vi "GUI_laptop v5.vi"() -> ()   [LabVIEW 2019]
uses:
  <vilib>/Platform/TimedLoop/XDataNode/timing_clust.ctl
  <vilib>/Platform/TimedLoop/XDataNode/nitl_modes.ctl
  <vilib>/Platform/TimedLoop/XDataNode/wakeup.ctl
  <vilib>/Instr/_visa.llb/VISA Configure Serial Port (Instr).vi
  <vilib>/Utility/file.llb/Write Delimited Spreadsheet (DBL).vi
  <vilib>/platform/TimedLoop/XDataNode/XDataNode.xnode
  <vilib>/Platform/TimedLoop/XDataNode/XDNodeRunTimeDep.lvlib
panel:
  out "Array - Numeric":dbl[](array[numeric])
  out "Num bytes received":i32
  in  "Joystick Type":dbl(ring) items=["Rigid Joystick", "Free Joystick"]
  out "Finished Late? [i-1]":bool
  out "Iteration Duration":i64
  in  "Stop":bool
  in  "Save  Data":bool
  in  "Save Path":path
  out "error out":errorcluster
  in  "baud rate":u32=115200
  in  "VISA resource name":refnum<visa-resource-name>
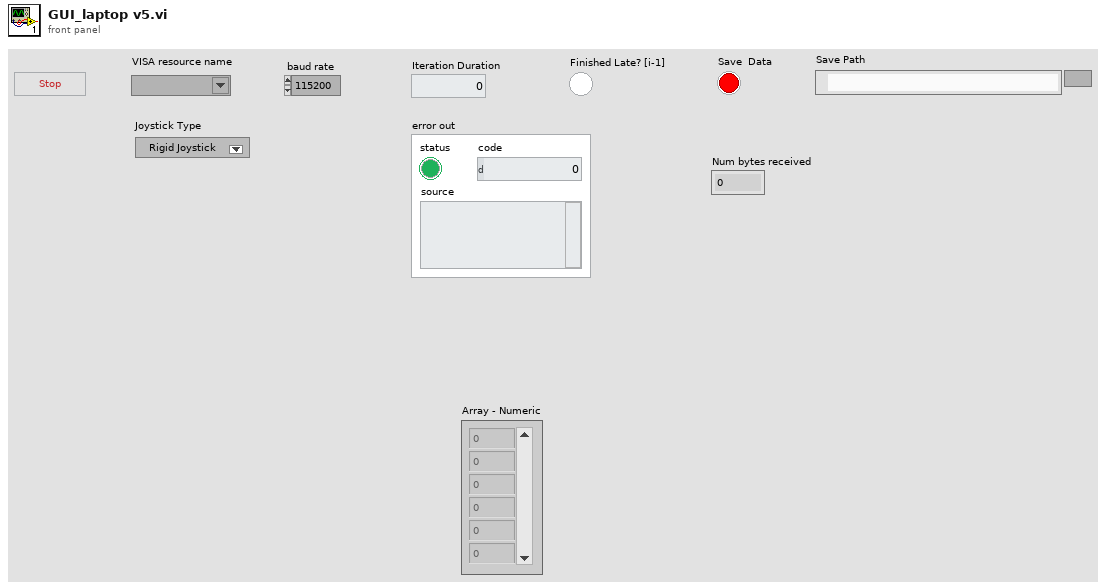
[diagram p1: front panel]
types:
  T1 = typedef "XDNodeRunTimeDep.lvlib/timing_clust.ctl" = cluster{"Expected End [f-1]":u64, "Actual End [f-1]":u64, "Finished Late? [f-1]":bool, "Expected End [i-1]":u64, "Actual End [i-1]":u64, "Finished Late? [i-1]":bool, "Expected Start [i]":u64, "Actual Start [i]":u64, "Expected Start [f]":u64, "Actual Start [f]":u64, "Source Name":string, "Structure Name":string, "Period":i64, "Deadline":i64, "Offset":i64, "Start":i64, "Priority":i32, "Timeout":i32, "Mode":T2, "Wakeup Reason":T3, "Error":errorcluster, "Source Type":string, "Secondary Source Type":string, "Global End Time":u64, "Global Start Time":u64, "Frame Duration":u64, "Iteration Duration":u64, "Assigned CPU":i32, "I/O Scan Engine Mode":u32}
  T2 = typedef "XDNodeRunTimeDep.lvlib/nitl_modes.ctl" = enum32{"No Change", "Process missed periods, maintain original phase", "Discard missed periods, maintain original phase", "Process missed periods, ignore original phase", "Discard missed periods, ignore original phase"}
  T3 = typedef "XDNodeRunTimeDep.lvlib/wakeup.ctl" = enum32{"Normal", "Aborted", "Asynchronous wakeup", "Timing source error", "Timed loop error", "Timeout"}
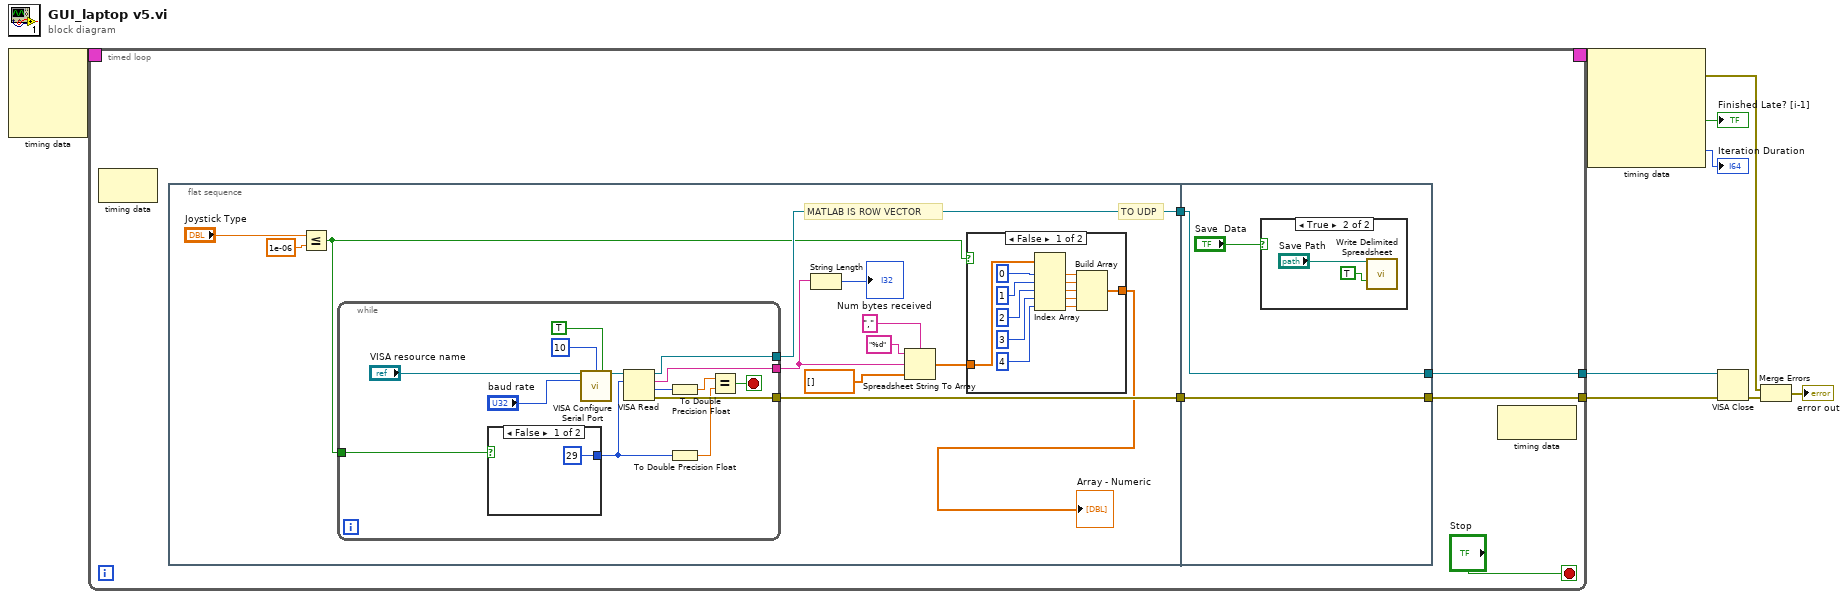
[diagram p0: block diagram]
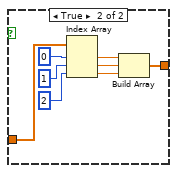
[diagram p2: hidden frame]
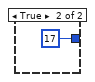
[diagram p3: hidden frame]
diagram:
  n1 = node-c288() -> (w9:T1)  [unwired: 4 in]
  n2 = timed-loop {
    tunnel: [w13] -> w7
    tunnel: [w12] -> w6
    timing: w9 -> [_]
    timing-out: [_] -> w8
    stop <- "Stop" stop-if-true
    n3 = node-c288() -> ()  [unwired: 1 in, 1 out]
    n4 = flat-sequence {
      tunnel: [w24] -> w11
      tunnel: [w26] -> w10
      tunnel: w11 -> [w67]
      tunnel: w10 -> [w66]
      tunnel: [w67] -> w13
      tunnel: [w66] -> w12
      frame #0 {
        # "TO UDP"
        # "MATLAB IS ROW VECTOR"
        n5 = Less Or Equal?(x="Joystick Type", y=1e-06) -> (x <= y?=w20:bool)
        n6 = while {
          tunnel: [w62] -> w19
          tunnel: [w58] -> w26
          tunnel: [w52] -> w24
          tunnel: w20 -> [w51]
          stop <- w61 stop-if-true
          n7 = case shown="False" w51 {
            tunnel: [29 u32 17 ("byte count")] -> w50
            frame False {
            }
            frame True {
            }
          }
          n8 = call-poly "VISA Configure Serial Port"("VISA resource name"="VISA resource name", "termination char\n(0xA = '\\n' = LF)"=u8 10 ("termination char\n(0xA = '\\n' = LF)"), "Enable Termination\nChar (T)"=TRUE ("Enable Termination\nChar (T)"), "baud rate (9600)"="baud rate") -> ("VISA resource name out"=w53:refnum<visa-resource-name>)  [unwired: 10 in, 1 out]
          n9 = VISA Read(VISA resource name=w53, byte count=w50) -> (VISA resource name out=w52:refnum<visa-resource-name>, read buffer=w62:string, return count=w60:u32, error out=w58:errorcluster)  [unwired: 1 in]
          n10 = To Double Precision Float(number=w60) -> (double precision float=w59:dbl)
          n11 = To Double Precision Float(number=w50) -> (double precision float=w49:dbl)
          n12 = Equal?(x=w59, y=w49) -> (x = y?=w61:bool)
        }
        n13 = String Length(string=w19) -> (length=→"Num bytes received":i32)
        n14 = Spreadsheet String To Array(delimiter (Tab)=",", format string="%d", spreadsheet string=w19, array type (2D Dbl)=dbl[] []) -> (array=w21:dbl[])
        n15 = case shown="False" w20 {
          tunnel: w21 -> [w29 w42]
          tunnel: [w34 w41] -> w17
          frame False {
            n16 = Index Array(array=w29, index #1=0 ("Plot ID"), index #2=1 ("Plot ID"), index #3=2 ("Plot ID"), index #4=3 ("Plot ID"), index #5=4 ("Plot ID")) -> (element #1=w37:dbl, element #2=w36:dbl, element #3=w35:dbl, element #4=w31:dbl, element #5=w30:dbl)
            n17 = Build Array(w37, w36, w35, w31, w30) -> (w34:dbl[])
          }
          frame True {
            n18 = Index Array(array=w42, index #1=0 ("Plot ID"), index #2=1 ("Plot ID"), index #3=2 ("Plot ID")) -> (element #1=w45:dbl, element #2=w44:dbl, element #3=w43:dbl)
            n19 = Build Array(w45, w44, w43) -> (w41:dbl[])
          }
        }
        "Array - Numeric" <- w17
      }
      frame #1 {
        n20 = case shown="True" "Save  Data" {
          frame False {
          }
          frame True {
            n21 = call-poly <vilib>:"Write Delimited Spreadsheet.vi"("file path (dialog if empty)"="Save Path", "append to file? (new file:F)"=TRUE) -> ()  [unwired: 12 in, 2 out]
          }
        }
      }
    }
    n22 = node-c288() -> ()  [unwired: 1 in, 1 out]
  }
  n23 = node-c288(w8) -> (w5:errorcluster, →"Finished Late? [i-1]":bool, →"Iteration Duration":i64)  [unwired: 3 out]
  n24 = VISA Close(VISA resource name=w7, error in (no error)=w6) -> (error out=w4:errorcluster)
  n25 = Merge Errors(w5, w4) -> (→"error out":errorcluster)
